vi "Main.vi"(11 "Module Admin":refnum<class "Delacor_lib_QMH_Module Admin.lvclass">) -> ()   [LabVIEW 2023, in "AutoPV.lvlib"]
doc: "This template is based off of the Queued Message Handler design pattern and the Queued Message Handler project template that ships with LabVIEW.\n\nThe main difference is that the queue is private to this module and communication between modules is performed via Broadcast and Request events.\n\nRequest events are wrapped in public API methods and are handled in the Event Handling Loop (EHL) of this VI. Any module can register for Broadcast events sent by this module. The EHL generates messages based on user interface actions.\n\nThe Message Handling Loop (MHL) processes messages generated by the EHL, or by other messages. The messages are string values, so new messages can be added easily to the Message Cases case structure in the MHL. Each message cluster can also provide an optional value for Message Data, which is a variant that can be converted to whatever message-specific data is required.\n_____\nBased on DQMH Project Template 6.1.0.94."
uses:
  AutoPV.lvlib
  <vilib>/Delacor/Delacor QMH/Libraries/Module Admin_class/Delacor_lib_QMH_Module Admin.lvclass
  Module Data--cluster.ctl
  <vilib>/ActorFramework/Message Enqueuer/Message Enqueuer.lvclass
  Drive/Pump_Data_Type.ctl
  Initial Data/InitalData Type.ctl
  Stop Argument--cluster.ctl
  <vilib>/Delacor/Delacor QMH/Libraries/Message Queue_class/Delacor_lib_QMH_Message Queue.lvclass/Delacor_lib_QMH_Message Queue.ctl
  <vilib>/Delacor/Delacor QMH/Libraries/Module Admin_class/Delacor_lib_QMH_Module Admin.lvclass/Delacor_lib_QMH_Module Admin.ctl
  Write_Dot Argument--cluster.ctl
  Update List UI Argument--cluster.ctl
  SubPanel Argument--cluster.ctl
  <vilib>/Utility/miscctls.llb/LVPointTypeDef.ctl
  Param_SL.ctl
  <vilib>/Delacor/Delacor QMH/Libraries/Message Queue_class/Delacor_lib_QMH_Enqueue Message (Single).vi
  <vilib>/Delacor/Delacor QMH/Libraries/Module Admin_class/Delacor_lib_QMH_Get External Launch.vi
  <vilib>/Analysis/baseanly.llb/Mean (DBL).vi
  <vilib>/Utility/file.llb/Read Delimited Spreadsheet (string).vi
  <vilib>/Utility/file.llb/Write Delimited Spreadsheet (string).vi
  <vilib>/Utility/error.llb/Error Cluster From Error Code.vi
  <vilib>/ErrorRing/Error Ring.xnode
  <vilib>/Delacor/Delacor QMH/Libraries/Message Queue_class/Delacor_lib_QMH_Message Queue.lvclass
  SFC/SFC.lvlib
  <vilib>/Kortex/Actor Planer/Actor Planer.lvlib
  <vilib>/Analysis/NI_AALBase.lvlib
  Drive/Drive.lvlib
  <vilib>/Utility/sysdir.llb/System Directory Type.ctl
  <vilib>/Utility/config.llb/NI_LVConfig.lvlib
  Initial Data/Initial Data.lvlib
  Dispatcher/Dispatcher.lvlib
panel:
  in  "Add 2":bool
  in  "Delete 2":bool
  in  "Save 2":bool
  in  "Load 2":bool
  in  "Архив экспериментов 2":bool
  in  "Add":bool
  in  "Pressure_edit":dbl=0.1 caption="Рредакт." min=0.1 max=99.99 format="%#.3f МПа"
  in  "Delete":bool
  in  "Save":bool
  in  "Load":bool
  in  "Pressure_List":i32(listbox) caption="Рзад, МПа"
  in  "Start":bool
  out "Time 2":dbl caption="Время отстоя" min=0.0 max=9999.0 format="%d сек."
  out "Mix_RPM 2":dbl=0.1 caption="Обороты мешалки" min=-1500.0 max=1500.0 format="%#.1f об\\мин"
  out "Stab_dP 2":dbl=0.1 caption="Стабилизация" min=0.1 max=20.0 format="%#.3f МПа"
  out "N 2":u32=1 caption="Текущая ступень" min=1 max=9999
  out "Stab_Time 2":dbl caption="Время перемешивания" min=0.0 max=9999.0 format="%d сек."
  out "dP 2":dbl=0.1 caption="Уставка давления" min=0.1 max=20.0 format="%#.2f МПа"
  out "P0 2":dbl=1.0 caption="Текущее давление" min=1.0 max=99.0 format="%#.2f МПа"
  in  "Time":dbl caption="Время отстоя" min=0.0 max=9999.0 format="%#.1f сек."
  in  "Mix_RPM":dbl=0.1 caption="Обороты мешалки" min=-1500.0 max=1500.0 format="%#.1f об\\мин"
  in  "Stab_dP":dbl=0.1 caption="Условие стабилизации" min=0.001 max=20.0 format="%#.3f МПа"
  in  "N":u32=1 caption="Кол-во ступеней" min=1 max=9999
  in  "Stab_Time":dbl caption="Время перемешивания" min=0.0 max=9999.0 format="%#.1f сек."
  out "relative seconds":dbl format="%_19f"
  in  "dP":dbl=0.1 caption="Шаг по давлению" min=0.01 max=20.0 format="%#.2f МПа"
  in  "P0":dbl=1.0 caption="Начальное давление" min=1.0 max=99.0 format="%#.2f МПа"
  in  "Pop-Out Tool 2":bool
  in  "Pop-Out Tool":bool
  out "PV-График":T1(graph)
  out "error out":errorcluster
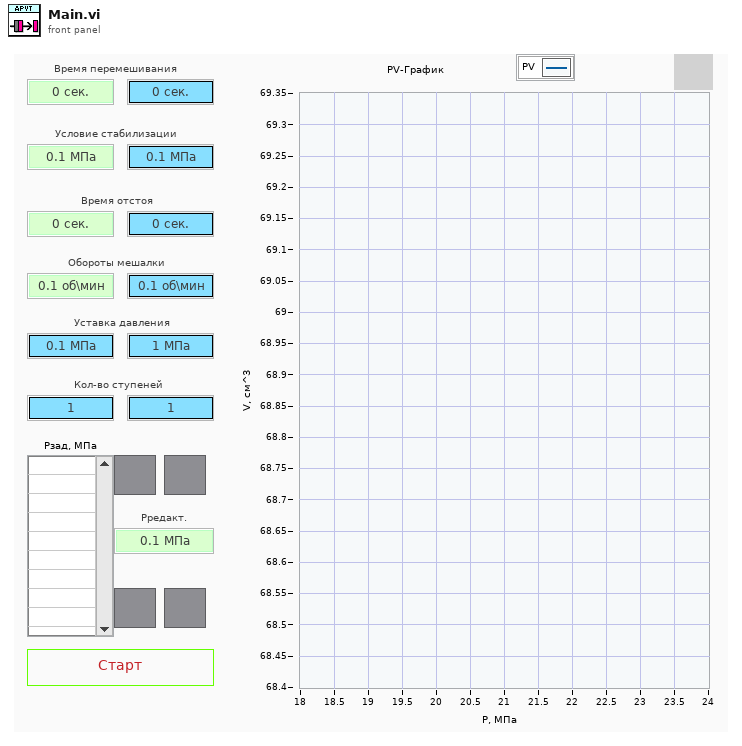
[diagram p1: front panel]
types:
  T1 = cluster{"Array - Dots":dbl[], "Array - Dots":dbl[]}
  T2 = typedef "Heat UI.lvlib/Broadcast Events--cluster.ctl" = cluster{"Module Did Init":refnum<user-event>, "Status Updated":refnum<user-event>, "Error Reported":refnum<user-event>, "Module Did Stop":refnum<user-event>, "Update Module Execution Status":refnum<user-event>, "T Data":refnum<user-event>, "Temp array":refnum<user-event>}
  T3 = typedef "Dispatcher.lvlib/Broadcast Events--cluster.ctl" = cluster{"Module Did Init":refnum<user-event>, "Status Updated":refnum<user-event>, "Error Reported":refnum<user-event>, "Module Did Stop":refnum<user-event>, "Update Module Execution Status":refnum<user-event>}
  T4 = typedef "Initial Data.lvlib/Broadcast Events--cluster.ctl" = cluster{"Module Did Init":refnum<user-event>, "Status Updated":refnum<user-event>, "Error Reported":refnum<user-event>, "Module Did Stop":refnum<user-event>, "Update Module Execution Status":refnum<user-event>, "Data":refnum<user-event>}
  T5 = typedef "Drive.lvlib/Broadcast Events--cluster.ctl" = cluster{"Module Did Init":refnum<user-event>, "Status Updated":refnum<user-event>, "Error Reported":refnum<user-event>, "Module Did Stop":refnum<user-event>, "Update Module Execution Status":refnum<user-event>, "Pump_Data":refnum<user-event>, "Rotate Data":refnum<user-event>, "Pump2 data":refnum<user-event>}
  T6 = typedef "AutoPV.lvlib/Request Events--cluster.ctl" = cluster{"Stop Module":refnum<user-event>, "Show Panel":refnum<user-event>, "Hide Panel":refnum<user-event>, "Get Module Execution Status":refnum<user-event>, "Show Diagram":refnum<user-event>, "Write_Dot":refnum<user-event>, "Update List UI":refnum<user-event>, "SubPanel":refnum<user-event>}
  T7 = typedef "SFC.lvlib/Control TypeDef.ctl" = cluster{"queue":refnum<queue>, "error":errorcluster, "Step":T8, "Algorythm":T8[]}
  T8 = typedef "SFC.lvlib/Step TypeDef.ctl" = cluster{"Name":string, "Timeout":dbl}
  T9 = typedef "AutoPV.lvlib/Module Data--cluster.ctl" = cluster{"Plan Enqueuer":refnum<class "Message Enqueuer.lvclass">, "Array P":dbl[], "Pump_data":T10, "Array - Dots":dbl[][], "Исходные данные":T11, "Temp array":dbl[], "Pressure_List ref":refnum<vi>, "Table select":i32, "PV_N":i32, "PV_N ref":refnum<vi>, "N ref":refnum<vi>, "Subpanel Ref":refnum<vi>}
  T10 = typedef "Drive.lvlib/Pump_Data_Type.ctl" = cluster{"Pressure PV":dbl, "Flow PV":dbl, "Volume PV":dbl, "Position_MM":dbl, "Volume corrected":dbl, "mix rpm":dbl}
  T11 = typedef "Initial Data.lvlib/InitalData Type.ctl" = cluster{"Дата":string, "Время":string, "Месторождение":string, "Пласт":string, "Скважина":string}
  T12 = enum32{"Invalid", "Standard", "Closed", "Hidden", "Minimized", "Maximized"}
  T13 = enum32{"invalid lock state", "Not Locked", "Locked (No Password)", "Password-protected"}
  T14 = typedef "AutoPV.lvlib/Stop Argument--cluster.ctl" = cluster{"Origin":string, "Exit via Stop Module Req?":bool, "Wait for Module to stop?":bool}
  T15 = typedef "AutoPV.lvlib/Write_Dot Argument--cluster.ctl" = cluster{"Clean?":bool, "Finish?":bool}
  T16 = typedef "AutoPV.lvlib/Update List UI Argument--cluster.ctl" = cluster{"Boolean":bool}
  T17 = typedef "AutoPV.lvlib/SubPanel Argument--cluster.ctl" = cluster{"Sub Panel":refnum<vi>}
  T18 = typedef "AutoPV.lvlib/Param_SL.ctl" = cluster{"P0":dbl, "dP":dbl, "Stab_Time":dbl, "N":u32, "Stab_dP":dbl, "Mix_RPM":dbl, "Time":dbl, "Item Names":string[]}
  T19 = typedef "LVPointTypeDef.ctl" = cluster{"Horizontal":i16, "Vertical":i16}
  T20 = typedef "NI_LVConfig.lvlib/Config Data RefNum.ctl" = refnum<k1>
  T21 = typedef "System Directory Type.ctl" = i32
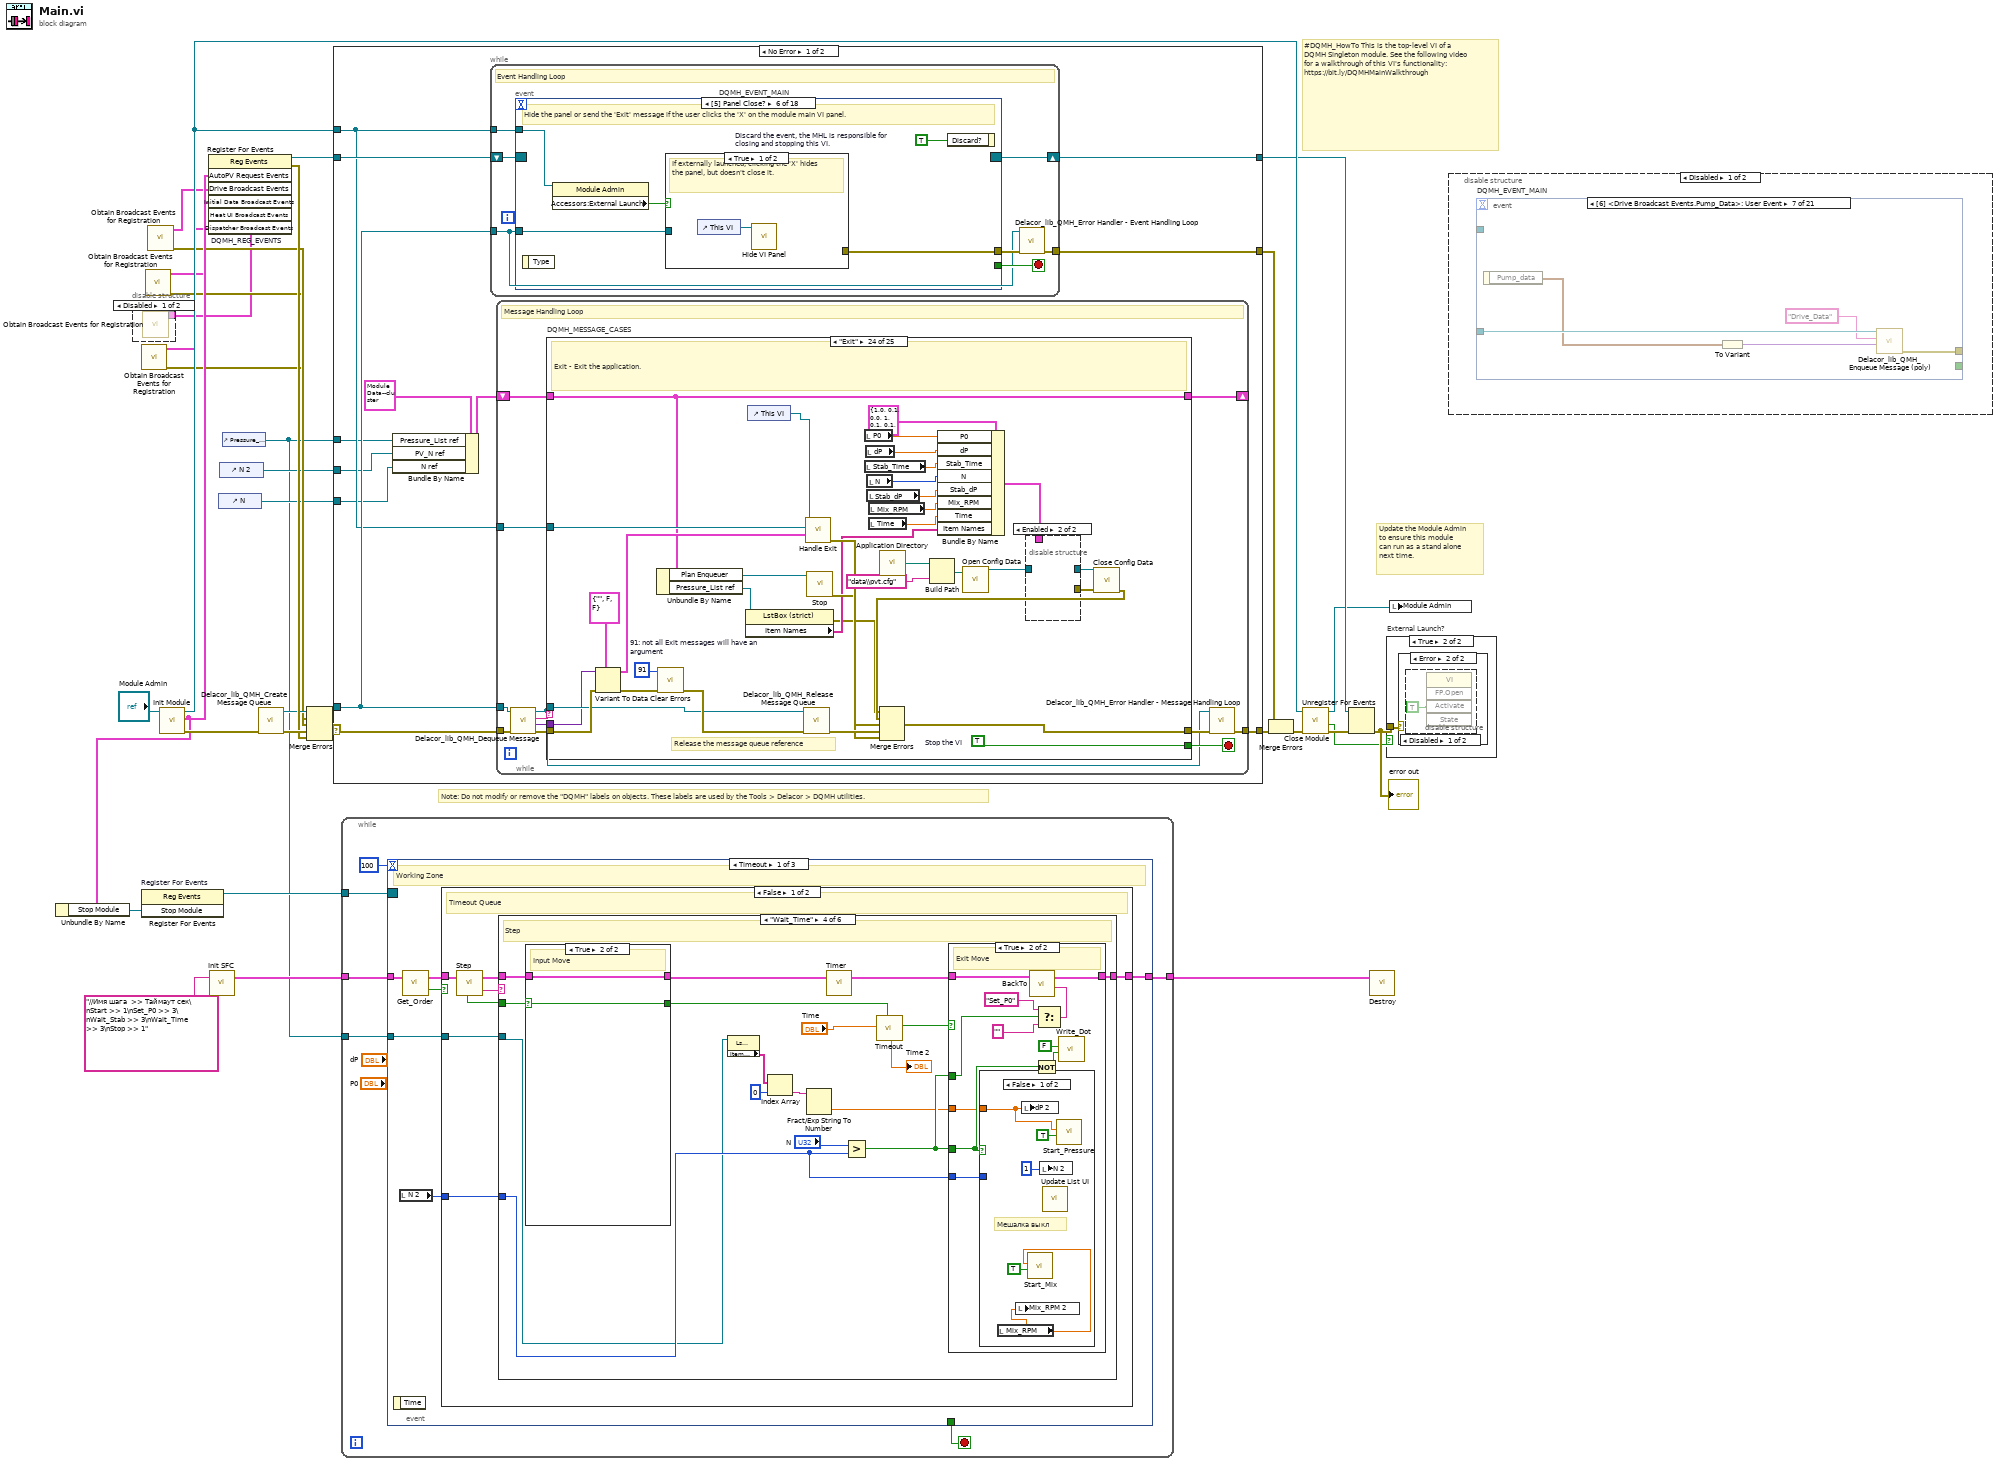
[diagram p0: block diagram]
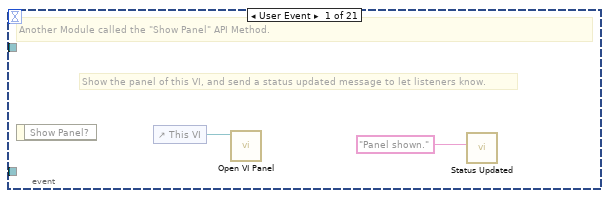
[diagram p2: hidden frame]
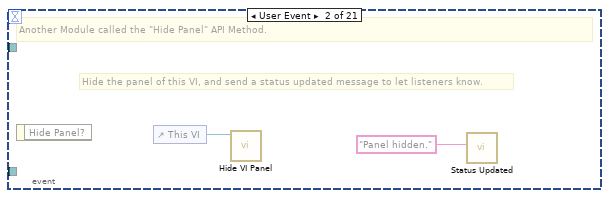
[diagram p3: hidden frame]
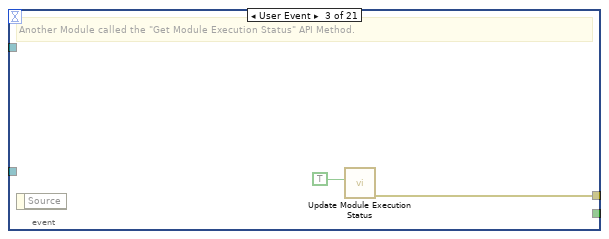
[diagram p4: hidden frame]
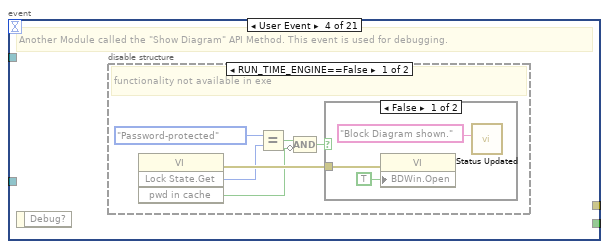
[diagram p5: hidden frame]
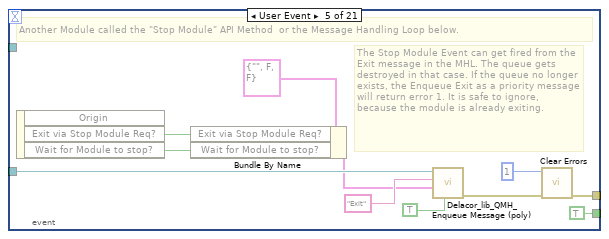
[diagram p8: hidden frame]
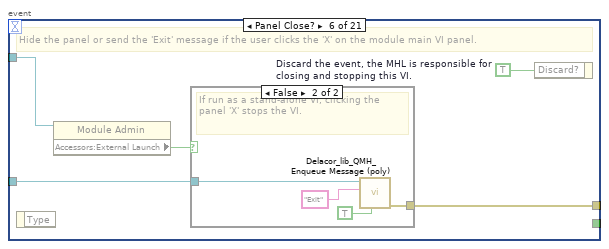
[diagram p9: hidden frame]
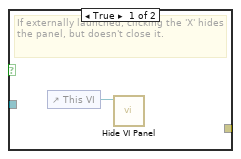
[diagram p10: hidden frame]
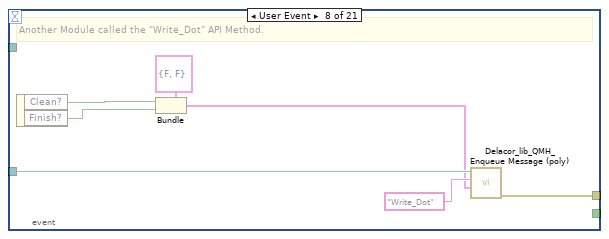
[diagram p11: hidden frame]
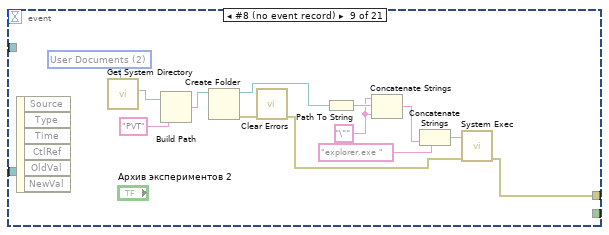
[diagram p12: hidden frame]
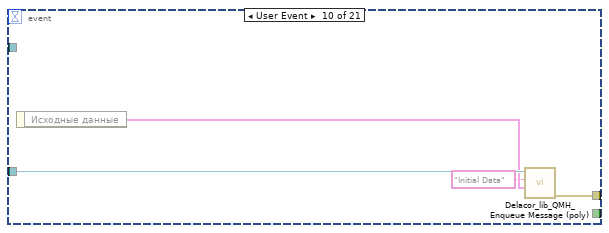
[diagram p13: hidden frame]
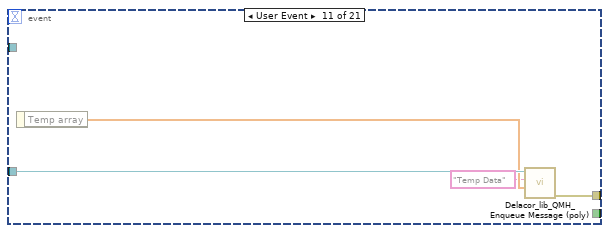
[diagram p14: hidden frame]
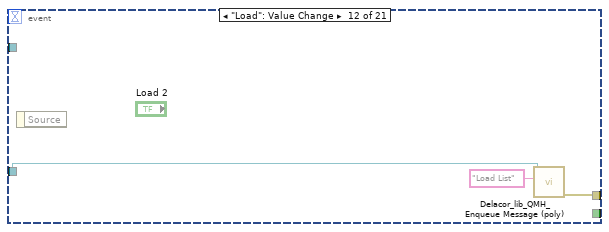
[diagram p15: hidden frame]
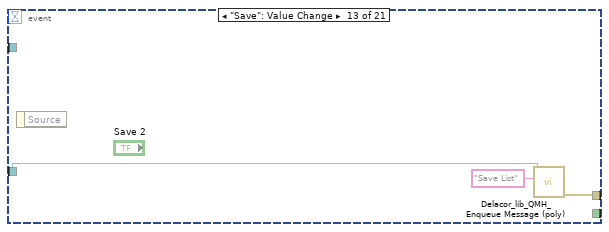
[diagram p16: hidden frame]
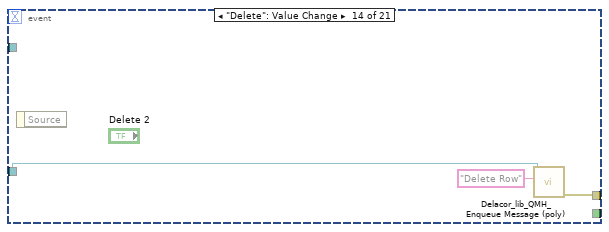
[diagram p17: hidden frame]
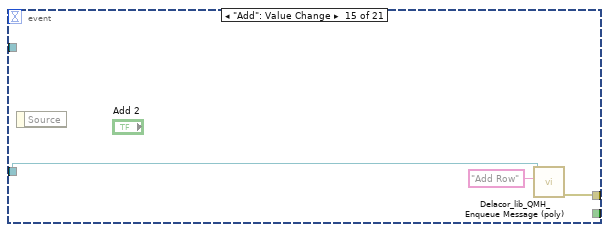
[diagram p18: hidden frame]
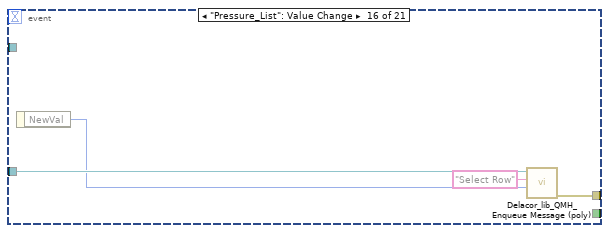
[diagram p19: hidden frame]
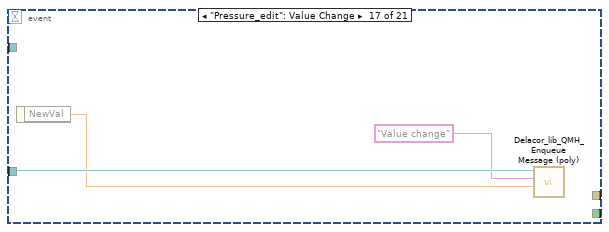
[diagram p20: hidden frame]
diagram:
  # "#DQMH_HowTo This is the top-level VI of a DQMH Singleton module. See the following video for a walkthrough of this VI's functionality: https://bit.ly/DQMHMainWalkthrough"
  # "Note: Do not modify or remove the \"DQMH\" labels on objects. These labels are used by the Tools > Delacor > DQMH utilities."
  # "Update the Module Admin to ensure this module can run as a stand alone next time."
  n1 = disable-structure shown="Disabled" {
    disable-tunnel: [w33 _] -> w6
    frame Disabled {
      n2 = call "Obtain Broadcast Events for Registration.vi"() -> ("Heat UI Broadcast Events"=w33:T2)  [unwired: 9 in, 2 out]
    }
    frame Enabled {
    }
  }
  n3 = call "Obtain Broadcast Events for Registration.vi"() -> ("error out"=w1:errorcluster, "Dispatcher Broadcast Events"=w2:T3)  [unwired: 9 in, 1 out]
  n4 = call "Obtain Broadcast Events for Registration.vi"() -> ("error out"=w7:errorcluster, "Initial Data Broadcast Events"=w8:T4)  [unwired: 9 in, 1 out]
  n5 = call "Obtain Broadcast Events for Registration.vi"() -> ("error out"=w9:errorcluster, "Drive Broadcast Events"=w10:T5)  [unwired: 9 in, 1 out]
  n6 = call "Init Module.vi"("Singleton Module Admin in"="Module Admin") -> ("error out"=w31:errorcluster, "AutoPV Request Events"=w12:T6, "Singleton Module Admin out"=w23:refnum<class "Delacor_lib_QMH_Module Admin.lvclass">)  [unwired: 8 in]
  n7 = Unbundle By Name(w12) -> ("Stop Module"=w11:refnum<user-event>)
  n8 = register-events "Register For Events"(w11) -> (reference out=w16:refnum<event-registration>)  [unwired: 2 in, 1 out]
  n9 = register-events "DQMH_REG_EVENTS"(w12, w10, w8, w6, w2) -> (reference out=w21:refnum<event-registration>, error out=w24:errorcluster)  [unwired: 2 in]
  n10 = call "Init SFC.vi"("Algo"="//Имя шага  >> Таймаут сек\nStart >> 1\nSet_P0 >> 3\nWait_Stab >> 3\nWait_Time >> 3\nStop >> 1") -> ("Control"=w15:T7)  [unwired: 18 in]
  n11 = control-ref of="N"() -> (w4:refnum<vi>)
  n12 = control-ref of="N 2"() -> (w5:refnum<vi>)
  n13 = control-ref of="Pressure_List"() -> (w3:refnum<vi>)
  n14 = call <vilib>:"Delacor_lib_QMH_Create Message Queue.vi"("error in"=w31) -> ("error out"=w26:errorcluster, "Message Queue"=w20:refnum<class "Delacor_lib_QMH_Message Queue.lvclass">)  [unwired: 9 in]
  n15 = Merge Errors(w1, w7, w9, w26, w24) -> (w25:errorcluster)
  n16 = case shown="No Error" w25 {
    selector: w25 -> [w43 w492]
    tunnel: [w45 w491] -> w32
    tunnel: [w42 w497] -> w22
    tunnel: w21 -> [w40 w497]
    tunnel: w20 -> [w39 w490]
    tunnel: [w44 _] -> w29
    tunnel: w23 -> [w38 w493]
    tunnel: w3 -> [w36 _]
    tunnel: w5 -> [w35 _]
    tunnel: w4 -> [w34 _]
    frame No Error {
      n17 = Bundle By Name(cluster=T9 {"Plan Enqueuer"=refnum, "Array P"=[], "Pump_data"={"Pressure PV"=0.0, "Flow PV"=0.0, "Volume PV"=0.0, "Position_MM"=0.0, "Volume corrected"=0.0, "mix rpm"=0.0}, "Array - Dots"=[], "Исходные данные"={"Дата"="", "Время"="", "Месторождение"="", "Пласт"="", "Скважина"=""}, "Temp array"=[], "Pressure_List ref"=refnum, "Table select"=0, "PV_N"=0, "PV_N ref"=refnum, "N ref"=refnum, "Subpanel Ref"=refnum} ("Data Cluster"), "Pressure_List ref"=w36, "PV_N ref"=w35, "N ref"=w34) -> (w37:T9)
      n18 = while {
        tunnel: w39 -> [w46]
        shift-right: [w49] -> w42
        shift-left: w40 -> [w50]
        tunnel: [w51] -> w44
        tunnel: w38 -> [w47]
        stop <- w48 stop-if-true
        # "Event Handling Loop"
        n19 = event "DQMH_EVENT_MAIN" shown="[5] Panel Close?" {
          selector: w50 -> [_ _ _ _ _ _ _ _ _ _ _ _ _ _ _ _ _ _]
          dyn-events: [_ _ _ _ _ _ _ _ _ _ _ _ _ _ _ _ _ _] -> w49
          timeout: _ -> [_ _ _ _ _ _ _ _ _ _ _ _ _ _ _ _ _ _]
          tunnel: [_ _ _ _ TRUE ("Discard?") _ _ _ _ _ _ _ _ _ _ _ _ _] -> w48
          tunnel: w46 -> [_ _ _ _ w76 w83 w94 w102 w106 w108 w111 w114 w117 w121 w125 w131 w137 w138]
          tunnel: [_ _ w60 _ w79 w85 w95 w97 w103 w109 w112 w115 w118 w122 _ w126 w132 w139] -> w52
          tunnel: w47 -> [_ _ _ _ _ w82 _ _ _ _ _ _ _ _ _ _ _ _]
          event User Event {
            # "Show the panel of this VI, and send a status updated message to let listeners know."
            # "Another Module called the \"Show Panel\" API Method."
            n20 = event-data() -> ()  [unwired: 1 in, 1 out]
            n21 = control-ref of="This VI"() -> (w54:refnum<vi>)
            n22 = call "Open VI Panel.vi"("VI"=w54) -> ()  [unwired: 10 in, 1 out]
            n23 = call "Status Updated.vi"("Status"="Panel shown." ("format string")) -> ()  [unwired: 10 in, 1 out]
          }
          event User Event {
            # "Hide the panel of this VI, and send a status updated message to let listeners know."
            # "Another Module called the \"Hide Panel\" API Method."
            n24 = event-data() -> ()  [unwired: 1 in, 1 out]
            n25 = control-ref of="This VI"() -> (w57:refnum<vi>)
            n26 = call "Hide VI Panel.vi"("VI"=w57) -> ()  [unwired: 10 in, 1 out]
            n27 = invoke class="VI" method="FP.Open"(reference=w57, "Activate"=FALSE ("Activate?"), "State"=T12."Closed") -> ()  [unwired: 2 in, 5 out]
            n28 = call "Status Updated.vi"("Status"="Panel hidden." ("format string")) -> ()  [unwired: 10 in, 1 out]
          }
          event User Event {
            # "Another Module called the \"Get Module Execution Status\" API Method."
            n29 = event-data() -> ()  [unwired: 1 in, 1 out]
            n30 = call "Update Module Execution Status.vi"("Running?"=TRUE) -> ("error out"=w60:errorcluster)  [unwired: 10 in]
          }
          event User Event {
            # "Another Module called the \"Show Diagram\" API Method. This event is used for debugging."
            n31 = event-data() -> ()  [unwired: 1 in, 1 out]
            n32 = disable-structure shown="RUN_TIME_ENGINE==False" {
              frame condition #0 (active) {
                # "functionality not available in exe"
                n33 = invoke class="VI" method="Lock State.Get"() -> (error out=w66:errorcluster, "Get Lock State"=w65:T13, "pwd in cache"=w62:bool)  [unwired: 4 in, 1 out]
                n34 = Equal?(x=T13."Password-protected", y=w65) -> (x = y?=w63:bool)
                n35 = Compound Arithmetic op=AND(w63, invert w62) -> (w61:bool)
                n36 = case shown="False" w61 {
                  tunnel: w66 -> [w69 _]
                  frame False {
                    n37 = property class="VI"(error in=w69, "BDWin.Open"=TRUE ("Block Diagram Window:Open")) -> ()  [unwired: 1 in, 2 out]
                    n38 = call "Status Updated.vi"("Status"="Block Diagram shown." ("format string")) -> ()  [unwired: 10 in, 1 out]
                  }
                  frame True {
                    # "Password-protected VI, and the password is not in the cache. Do not show the diagram."
                  }
                }
              }
              frame condition #1 {
              }
            }
          }
          event User Event {
            # "The Stop Module Event can get fired from the Exit message in the MHL. The queue gets destroyed in that case. If the queue no longer exists, the Enqueue Exit as a priority message will return error 1. It is safe to ignore, because the module is already exiting."
            # "Another Module called the \"Stop Module\" API Method  or the Message Handling Loop below."
            n39 = event-data() -> ("Exit via Stop Module Req?"=w72:bool, "Wait for Module to stop?"=w71:bool)  [unwired: 1 in, 1 out]
            n40 = Bundle By Name(cluster=T14 {"Origin"="", "Exit via Stop Module Req?"=FALSE, "Wait for Module to stop?"=FALSE} ("Stop Argument"), "Exit via Stop Module Req?"=w72, "Wait for Module to stop?"=w71) -> (w70:T14)
            n41 = call-poly <vilib>:"Delacor_lib_QMH_Enqueue Message (poly).vi"("Priority Message? (F)"=TRUE, "Message Data"=w70, "Message"="Exit", "Message Queue in"=w76) -> ("error out"=w80:errorcluster)  [unwired: 6 in, 1 out]
            n42 = call <vilib>:"Clear Errors.vi"("error in (no error)"=w80, "specific error code to clear (0: all)"=1) -> ("error out"=w79:errorcluster)  [unwired: 4 in, 1 out]
          }
          event Panel Close? {
            w84 = TRUE  # Discard the event, the MHL is responsible for closing and stopping this VI.
            # "Hide the panel or send the 'Exit' message if the user clicks the 'X' on the module main VI panel."
            n43 = event-data() -> ()  [unwired: 1 in, 1 out]
            n44 = property class="Module Admin"(reference=w82) -> ("Accessors:External Launch"=w81:bool)  [unwired: 1 in, 2 out]
            n45 = case shown="True" w81 {
              tunnel: w83 -> [_ w89]
              tunnel: [_ w90] -> w85
              frame True {
                # "If externally launched, clicking the 'X' hides the panel, but doesn't close it."
                n46 = control-ref of="This VI"() -> (w86:refnum<vi>)
                n47 = call "Hide VI Panel.vi"("VI"=w86) -> ()  [unwired: 10 in, 1 out]
              }
              frame False {
                # "If run as a stand-alone VI, clicking the panel 'X' stops the VI."
                n48 = call-poly <vilib>:"Delacor_lib_QMH_Enqueue Message (poly).vi"("Priority Message? (F)"=TRUE, "Message"="Exit", "Message Queue in"=w89) -> ("error out"=w90:errorcluster)  [unwired: 7 in, 1 out]
              }
            }
            n49 = event-data("Discard?"=w84) -> ()  [unwired: 1 in, 1 out]
          }
          event User Event {
            n50 = event-data() -> ("Pump_data"=w93:T10)  [unwired: 1 in]
            n51 = To Variant(anything=w93) -> (Variant=w91:variant)
            n52 = call-poly <vilib>:"Delacor_lib_QMH_Enqueue Message (poly).vi"("Message Data"=w91, "Message"="Drive_Data", "Message Queue in"=w94) -> ("error out"=w95:errorcluster)  [unwired: 7 in, 1 out]
          }
          event User Event {
            # "Another Module called the \"Write_Dot\" API Method."
            n53 = event-data() -> ("Clean?"=w98:bool, "Finish?"=w96:bool)  [unwired: 1 in]
            n54 = Bundle(cluster=T15 {"Clean?"=FALSE, "Finish?"=FALSE} ("Write_Dot Argument"), "Clean?"=w98, "Finish?"=w96) -> (w99:T15)
            n55 = call-poly <vilib>:"Delacor_lib_QMH_Enqueue Message (poly).vi"("Message Data"=w99, "Message"="Write_Dot", "Message Queue in"=w102) -> ("error out"=w97:errorcluster)  [unwired: 7 in, 1 out]
          }
          event User Event {
            n56 = event-data() -> ("Исходные данные"=w105:T11)  [unwired: 1 in]
            n57 = call-poly <vilib>:"Delacor_lib_QMH_Enqueue Message (poly).vi"("Message Data"=w105, "Message"="Initial Data", "Message Queue in"=w106) -> ("error out"=w103:errorcluster)  [unwired: 7 in, 1 out]
          }
          event "Load": Value Change {
            n58 = event-data() -> ()  [unwired: 1 in, 1 out]
            n59 = call-poly <vilib>:"Delacor_lib_QMH_Enqueue Message (poly).vi"("Message"="Load List", "Message Queue in"=w108) -> ("error out"=w109:errorcluster)  [unwired: 8 in, 1 out]
          }
          event "Save": Value Change {
            n60 = event-data() -> ()  [unwired: 1 in, 1 out]
            n61 = call-poly <vilib>:"Delacor_lib_QMH_Enqueue Message (poly).vi"("Message"="Save List", "Message Queue in"=w111) -> ("error out"=w112:errorcluster)  [unwired: 8 in, 1 out]
          }
          event "Delete": Value Change {
            n62 = event-data() -> ()  [unwired: 1 in, 1 out]
            n63 = call-poly <vilib>:"Delacor_lib_QMH_Enqueue Message (poly).vi"("Message"="Delete Row", "Message Queue in"=w114) -> ("error out"=w115:errorcluster)  [unwired: 8 in, 1 out]
          }
          event "Add": Value Change {
            n64 = event-data() -> ()  [unwired: 1 in, 1 out]
            n65 = call-poly <vilib>:"Delacor_lib_QMH_Enqueue Message (poly).vi"("Message"="Add Row", "Message Queue in"=w117) -> ("error out"=w118:errorcluster)  [unwired: 8 in, 1 out]
          }
          event "Pressure_List": Value Change {
            n66 = event-data() -> ("NewVal"=w120:i32)  [unwired: 1 in]
            n67 = call-poly <vilib>:"Delacor_lib_QMH_Enqueue Message (poly).vi"("Message Data"=w120, "Message"="Select Row", "Message Queue in"=w121) -> ("error out"=w122:errorcluster)  [unwired: 7 in, 1 out]
          }
          event "Pressure_edit": Value Change {
            n68 = event-data() -> ("NewVal"=w124:dbl)  [unwired: 1 in]
            n69 = call-poly <vilib>:"Delacor_lib_QMH_Enqueue Message (poly).vi"("Message Data"=w124, "Message"="Value change", "Message Queue in"=w125) -> ()  [unwired: 7 in, 2 out]
          }
          event User Event {
            # "Another Module called the \"Update List UI\" API Method."
            n70 = event-data() -> ("Boolean"=w127:bool)  [unwired: 1 in]
            n71 = Bundle(cluster=T16 {"Boolean"=FALSE} ("Update List UI Argument"), "Boolean"=w127) -> (w128:T16)
            n72 = call-poly <vilib>:"Delacor_lib_QMH_Enqueue Message (poly).vi"("Message Data"=w128, "Message"="Update List UI", "Message Queue in"=w131) -> ("error out"=w126:errorcluster)  [unwired: 7 in, 1 out]
          }
          event User Event {
            # "Another Module called the \"SubPanel\" API Method."
            n73 = event-data() -> ("Sub Panel"=w133:refnum<vi>)  [unwired: 1 in]
            n74 = Bundle(cluster=T17 {"Sub Panel"=refnum} ("SubPanel Argument"), "Sub Panel"=w133) -> (w134:T17)
            n75 = call-poly <vilib>:"Delacor_lib_QMH_Enqueue Message (poly).vi"("Message Data"=w134, "Message"="SubPanel", "Message Queue in"=w137) -> ("error out"=w132:errorcluster)  [unwired: 7 in, 1 out]
          }
          event "Pop-Out Tool": Value Change {
            n76 = event-data() -> ()  [unwired: 1 in, 2 out]
            n77 = call-poly <vilib>:"Delacor_lib_QMH_Enqueue Message (poly).vi"("Message"="Window", "Message Queue in"=w138) -> ("error out"=w139:errorcluster)  [unwired: 8 in, 1 out]
          }
        }
        n78 = call-dynamic "Delacor_lib_QMH_Error Handler - Event Handling Loop.vi"("error in"=w52, "Message Queue in"=w46) -> ("dup error in"=w51:errorcluster)  [unwired: 8 in, 1 out]
      }
      n79 = while {
        tunnel: w39 -> [w143]
        shift-right: [w147] -> _
        shift-left: w37 -> [w148]
        tunnel: w43 -> [w151]
        tunnel: [w149] -> w45
        tunnel: w38 -> [w141]
        stop <- w146 stop-if-true
        # "Message Handling Loop"
        n80 = call-dynamic "Delacor_lib_QMH_Dequeue Message.vi"("error in"=w151, "Message Queue in"=w143) -> ("error out"=w150:errorcluster, "Message Data"=w144:variant, "Message"=w145:string, "Message Queue out"=w142:refnum<class "Delacor_lib_QMH_Message Queue.lvclass">)  [unwired: 6 in]
        n81 = case "DQMH_MESSAGE_CASES" shown="\"Exit\"" w145 {
          selector: w145 -> [_ _ _ _ _ _ _ _ _ _ _ _ _ _ _ _ _ _ _ _ _ _ _ _ w477]
          tunnel: w142 -> [w161 _ w191 _ _ _ _ _ _ _ _ _ _ _ _ _ _ w370 _ _ _ _ w422 w465 _]
          tunnel: w150 -> [w185 w188 w205 w219 w227 w243 w256 w262 w273 w276 w285 w292 w300 w309 w316 w323 w340 w375 w392 w405 w407 w412 w429 w471 w479]
          tunnel: [w171 w188 w193 w214 w222 w240 w252 w261 w266 w275 w284 w291 w299 w308 w315 w322 w339 w382 w394 w404 w407 w411 w425 w468 w480] -> w152
          tunnel: w148 -> [w156 w187 w197 w215 w223 w238 w250 w258 w272 w274 w283 w290 w298 w306 w314 w321 w324 w381 w393 w400 w406 w409 w424 w457 w478]
          tunnel: [w176 w187 w199 w216 w224 w238 w253 w257 w264 w274 w283 w289 w297 w306 w314 w321 w324 w381 w389 w400 w406 w409 w424 w457 w478] -> w147
          tunnel: [_ _ _ _ _ _ _ _ _ _ _ _ _ _ _ _ _ _ _ _ _ _ _ w464 _] -> w146
          tunnel: w144 -> [_ _ w203 w217 w225 w241 w254 w260 w270 _ _ _ _ _ _ _ _ w374 w391 _ _ _ w423 w463 _]
          tunnel: w141 -> [w177 _ _ _ _ _ _ _ _ _ _ _ _ _ _ _ _ _ _ _ _ _ w421 w458 _]
          frame "Initialize" {
            w164 = T19 {"Horizontal"=0, "Vertical"=0} ("Origin")
            # "Initialize - Any operation that needs to be done before the module can receive messages. Synchronize Caller Events.vi will inform Start Module.vi that the module has launched and is ready to receive messages. Module Did Init.vi will broadcast that the module initialized."
            n82 = call "Synchronize Caller Events.vi"("error in (no error)"=w185, "Singleton Module Admin in"=w177) -> ("error out"=w184:errorcluster, "Singleton Module Admin out"=w173:refnum<class "Delacor_lib_QMH_Module Admin.lvclass">)  [unwired: 8 in]
            n83 = Unbundle By Name(w156) -> ("Pressure_List ref"=w155:refnum<vi>)
            n84 = property class="Module Admin"(reference=w173) -> ("Accessors:External Launch"=w181:bool)  [unwired: 1 in, 2 out]
            n85 = call <vilib>:"Start.vi"("DQMH Queue"=w161) -> ("error out"=w170:errorcluster, "Plan Enqueuer"=w169:refnum<class "Message Enqueuer.lvclass">)  [unwired: 9 in]
            n86 = property class="LstBox (strict)"(reference=w155, "Value"=-1) -> (error out=w154:errorcluster)  [unwired: 1 in, 1 out]
            n87 = Select(t=T12."Hidden" ("State"), s=w181, f=T12."Standard" ("State")) -> (s? t:f=w178:T12)
            n88 = call <vilib>:"Add Event.vi"("Continius? (F)"=TRUE, "Timeout (1 sec)"=1.0, "error in"=w170, "Action"="Stab" ("Message"), "Plan Enqueuer"=w169) -> ("error out"=w167:errorcluster, "Plan Enqueuer out"=w168:refnum<class "Message Enqueuer.lvclass">)  [unwired: 4 in, 1 out]
            n89 = property class="VI"("Front Panel.Title"="PV-кривая" ("Front Panel Window:Title")) -> (reference out=w182:refnum<vi>, error out=w186:errorcluster)  [unwired: 2 in]
            n90 = call "Module Name--constant.vi"() -> ("Module Name"=w174:string)  [unwired: 11 in]
            n91 = invoke class="VI" method="FP.Open"(reference=w182, error in=w186, "State"=w178) -> ()  [unwired: 2 in, 5 out]
            n92 = call "Module Did Init.vi"("error in (no error)"=w184, "Initialized?"=TRUE, "Origin"=w174) -> ("error out"=w183:errorcluster)  [unwired: 8 in]
            n93 = property on="Pane" class="Pane"("Position"=w164) -> ()  [unwired: 2 in, 2 out]
            n94 = property on="Pane 2" class="Pane"("Position"=w164) -> ()  [unwired: 2 in, 2 out]
            n95 = call-poly <vilib>:"Delacor_lib_QMH_Enqueue Message (poly).vi"("Message"="Load", "Message Queue in"=w161) -> ("error out"=w162:errorcluster)  [unwired: 8 in, 1 out]
            n96 = Merge Errors(w162, w167, w183, w154) -> (w171:errorcluster)
            n97 = Bundle By Name(cluster=w156, "Plan Enqueuer"=w168, "Table select"=-1, "PV_N"=0) -> (w176:T9)
            n98 = local write "Pressure_edit"(0.0 ("Pressure_edit")) -> ()
          }
          frame "---Module Specific---" {
            # "Separator -- The following cases handle messages specific to this Module."
          }
          frame "Write_Dot" {
            n99 = Unbundle By Name(w197) -> ("Array - Dots"=w196:dbl[][], "Pump_data.Pressure PV"=w195:dbl, "Pump_data.Volume corrected"=w194:dbl)
            n100 = Variant To Data(error in=w205, type=T15 {"Clean?"=FALSE, "Finish?"=FALSE} ("Write_Dot Argument"), Variant=w203) -> (data=w201:T15, error out=w204:errorcluster)
            n101 = Unbundle By Name(w201) -> ("Clean?"=w200:bool, "Finish?"=w189:bool)
            n102 = case shown="False" w200 {
              tunnel: [w209 dbl[][] [] ("Array - Dots")] -> w198
              tunnel: w196 -> [w210 _]
              tunnel: w195 -> [w208 _]
              tunnel: w194 -> [w207 _]
              frame False {
                n103 = Build Array(w208, w207) -> (w206:dbl[])
                n104 = Build Array (concatenate)(w210, w206) -> (w209:dbl[][])
              }
              frame True {
              }
            }
            n105 = Bundle By Name(cluster=w197, "Array - Dots"=w198) -> (w199:T9)
            n106 = call-poly <vilib>:"Delacor_lib_QMH_Enqueue Message (poly).vi"("Message Data"=w189, "Message"="Update Graph", "Message Queue in"=w191) -> ("error out"=w192:errorcluster)  [unwired: 7 in, 1 out]
            n107 = Merge Errors(w192, w204) -> (w193:errorcluster)
          }
          frame "Initial Data" {
            n108 = Variant To Data(error in=w219, type=T11 {"Дата"="", "Время"="", "Месторождение"="", "Пласт"="", "Скважина"=""} ("Исходные данные"), Variant=w217) -> (data=w212:T11, error out=w218:errorcluster)
            n109 = Bundle By Name(cluster=w215, "Исходные данные"=w212) -> (w216:T9)
            n110 = Merge Errors(w218) -> (w214:errorcluster)
          }
          frame "Temp Data" {
            n111 = Variant To Data(error in=w227, type=dbl[] [] ("Temp array"), Variant=w225) -> (data=w221:dbl[], error out=w226:errorcluster)
            n112 = Bundle By Name(cluster=w223, "Temp array"=w221) -> (w224:T9)
            n113 = Merge Errors(w226) -> (w222:errorcluster)
          }
          frame "Value change" {
            n114 = Variant To Data(error in=w243, type=0.0 ("NewVal"), Variant=w241) -> (data=w233:dbl, error out=w242:errorcluster)
            n115 = Unbundle By Name(w238) -> ("Pressure_List ref"=w237:refnum<vi>, "Table select"=w235:i32)
            n116 = Number To Fractional String(number=w233, precision (6)=i16 2) -> (F-format string=w232:string)  [unwired: 2 in]
            n117 = property class="LstBox (strict)"(reference=w237) -> (reference out=w231:refnum<vi>, error out=w230:errorcluster, "Item Names"=w236:string[])  [unwired: 1 in]
            n118 = Replace Array Subset(array=w236, new element=w232, index=w235) -> (w229:string[])
            n119 = property class="LstBox (strict)"(reference=w231, error in=w230, "Item Names"=w229) -> (error out=w228:errorcluster)  [unwired: 1 out]
            n120 = Merge Errors(w228, w242) -> (w240:errorcluster)
          }
          frame "Select Row" {
            n121 = Variant To Data(error in=w256, type="Pressure_List", Variant=w254) -> (data=w247:i32, error out=w255:errorcluster)
            n122 = Unbundle By Name(w250) -> ("Pressure_List ref"=w249:refnum<vi>)
            n123 = property class="LstBox (strict)"(reference=w249) -> (error out=w246:errorcluster, "Item Names"=w248:string[])  [unwired: 1 in, 1 out]
            n124 = Bundle By Name(cluster=w250, "Table select"=w247) -> (w253:T9)
            n125 = Index Array(array=w248, index=w247) -> (element=w245:string)
            n126 = Merge Errors(w246, w255) -> (w252:errorcluster)
            n127 = Fract/Exp String To Number(string=w245) -> (number=w244:dbl)  [unwired: 3 in, 1 out]
            n128 = local write "Pressure_edit"(w244) -> ()
          }
          frame "Update List UI" {
            n129 = Variant To Data(error in=w262, type=T16 {"Boolean"=FALSE} ("Update List UI Argument"), Variant=w260) -> (error out=w261:errorcluster)  [unwired: 1 out]
            n130 = call "Update UI List.vi"("Data Cluster"=w258) -> ("Data Cluster 2"=w257:T9)  [unwired: 9 in, 1 out]
          }
          frame "SubPanel" {
            n131 = Variant To Data(error in=w273, type=T17 {"Sub Panel"=refnum} ("SubPanel Argument"), Variant=w270) -> (data=w268:T17, error out=w271:errorcluster)
            n132 = Unbundle By Name(w268) -> ("Sub Panel"=w263:refnum<vi>)
            n133 = control-ref of="This VI"() -> (w267:refnum<vi>)
            n134 = call "Insert SubPanel.vi"("VI Ref"=w267, "Subpanel Ref"=w263) -> ("error out"=w265:errorcluster)  [unwired: 9 in]
            n135 = Bundle By Name(cluster=w272, "Subpanel Ref"=w263) -> (w264:T9)
            n136 = Merge Errors(w265, w271) -> (w266:errorcluster)
          }
          frame "---Copy This Frame---" {
            # "Duplicate this frame when creating new messages.  Change this comment in the duplicated frame to describe this message."
            n137 = Merge Errors(w276) -> (w275:errorcluster)
          }
          frame "Window" {
            # "Duplicate this frame when creating new messages.  Change this comment in the duplicated frame to describe this message."
            n138 = Unbundle By Name(w283) -> ("Subpanel Ref"=w278:refnum<vi>)
            n139 = control-ref of="This VI"() -> (w281:refnum<vi>)
            n140 = invoke class="SubPnl" method="Remove VI"(reference=w278) -> (error out=w279:errorcluster)  [unwired: 2 in, 2 out]
            n141 = invoke class="VI" method="FP.Close"(reference=w281, error in=w279) -> (reference out=w282:refnum<vi>)  [unwired: 1 in, 2 out]
            n142 = invoke class="VI" method="FP.Open"(reference=w282, "State"=T12."Standard") -> (error out=w277:errorcluster)  [unwired: 3 in, 4 out]
            n143 = Merge Errors(w277, w285) -> (w284:errorcluster)
          }
          frame "Add Row" {
            # "Duplicate this frame when creating new messages.  Change this comment in the duplicated frame to describe this message."
            n144 = call "Add row item.vi"("SP P"="Pressure_edit", "Data Cluster in"=w290) -> ("error out"=w288:errorcluster, "Data Cluster out"=w289:T9)  [unwired: 8 in]
            n145 = call "Update List UI.vi"() -> ("error out"=w286:errorcluster)  [unwired: 11 in]
            n146 = Merge Errors(w286, w288, w292) -> (w291:errorcluster)
          }
          frame "Delete Row" {
            # "Duplicate this frame when creating new messages.  Change this comment in the duplicated frame to describe this message."
            n147 = call "Delete row item.vi"("Data Cluster in"=w298) -> ("error out"=w296:errorcluster, "Ok?"=w294:bool, "New P"=w293:dbl, "Data Cluster out"=w297:T9)  [unwired: 7 in]
            n148 = call "Update List UI.vi"() -> ("error out"=w295:errorcluster)  [unwired: 11 in]
            n149 = case shown="True" w294 {
              tunnel: w293 -> [_ w301]
              frame False {
              }
              frame True {
                n150 = local write "Pressure_edit"(w301) -> ()
              }
            }
            n151 = Merge Errors(w295, w296, w300) -> (w299:errorcluster)
          }
          frame "Load List" {
            # "Duplicate this frame when creating new messages.  Change this comment in the duplicated frame to describe this message."
            n152 = Unbundle By Name(w306) -> ("Pressure_List ref"=w305:refnum<vi>)
            n153 = call-poly <vilib>:"Read Delimited Spreadsheet.vi"() -> ("first row"=w302:string[], "error out"=w307:errorcluster)  [unwired: 10 in, 4 out]
            n154 = property class="LstBox (strict)"(reference=w305, "Item Names"=w302) -> (error out=w304:errorcluster)  [unwired: 1 in, 1 out]
            n155 = call "Update List UI.vi"() -> ("error out"=w303:errorcluster)  [unwired: 11 in]
            n156 = Merge Errors(w303, w304, w307, w309) -> (w308:errorcluster)
          }
          frame "Save List" {
            # "Duplicate this frame when creating new messages.  Change this comment in the duplicated frame to describe this message."
            n157 = Unbundle By Name(w314) -> ("Pressure_List ref"=w313:refnum<vi>)
            n158 = property class="LstBox (strict)"(reference=w313) -> (error out=w312:errorcluster, "Item Names"=w311:string[])  [unwired: 1 in, 1 out]
            n159 = call-poly <vilib>:"Write Delimited Spreadsheet.vi"("1D data"=w311) -> ("error out"=w310:errorcluster)  [unwired: 13 in, 1 out]
            n160 = Merge Errors(w312, w310, w316) -> (w315:errorcluster)
          }
          frame "Save Report" {
            # "Duplicate this frame when creating new messages.  Change this comment in the duplicated frame to describe this message."
            n161 = Unbundle By Name(w321) -> ("Исходные данные"=w320:T11, "Temp array"=w318:dbl[], "Array - Dots"=w317:dbl[][])
            n162 = call "Save Report.vi"("Array - Dots"=w317, "Temp array"=w318, "Исходные данные"=w320) -> ("error out"=w319:errorcluster)  [unwired: 8 in]
            n163 = Merge Errors(w319, w323) -> (w322:errorcluster)
          }
          frame "Load" {
            # "Duplicate this frame when creating new messages.  Change this comment in the duplicated frame to describe this message."
            n164 = call <vilib>:"Application Directory.vi"() -> ("Application Directory"=w334:path)
            n165 = Unbundle By Name(w324) -> ("Pressure_List ref"=w327:refnum<vi>)
            n166 = Build Path(base path=w334, name or relative path="data\\pvt.cfg" ("string")) -> (appended path=w332:path)
            n167 = call <vilib>:"Open Config Data.vi"("configuration file path"=w332) -> ("error out"=w335:errorcluster, "file created?"=w338:bool, "refnum"=w337:T20)  [unwired: 8 in]
            n168 = case shown="False" w338 {
              tunnel: w337 -> [w357 w368]
              tunnel: T18 {"P0"=1.0, "dP"=0.1, "Stab_Time"=0.0, "N"=1, "Stab_dP"=0.1, "Mix_RPM"=0.1, "Time"=0.0, "Item Names"=[]} ("Cluster") -> [w354 _]
              tunnel: w335 -> [w345 w367]
              tunnel: [w356 _] -> w331
              tunnel: [w345 w367] -> w330
              tunnel: [w344 w368] -> w329
              tunnel: w327 -> [w343 w365]
              tunnel: [w341 w366] -> w326
              frame False {
                n169 = disable-structure shown="Disabled" {
                  disable-tunnel: w357 -> [w363 _]
                  disable-tunnel: [w362 _] -> w356
                  disable-tunnel: [w361 _] -> w355
                  disable-tunnel: w354 -> [w360 _]
                  disable-tunnel: w345 -> [w359 _]
                  disable-tunnel: [w358 _] -> w344
                  frame Disabled {
                    n170 = call <userlib>:"Read INI Cluster__ogtk.vi"("error in (no error)"=w359, "INI Fomatted Cluster Type"=w360, "refnum"=w363) -> ("error out"=w362:errorcluster, "INI Fomatted Cluster"=w361:variant, "dup refnum"=w358:T20)  [unwired: 4 in, 2 out]
                  }
                  frame Enabled {
                  }
                }
                n171 = Variant To Data(error in=w356, type=w354, Variant=w355) -> (data=w353:T18)  [unwired: 1 out]
                n172 = Unbundle By Name(w353) -> ("Item Names"=w342:string[], "P0"=w352:dbl, "dP"=w351:dbl, "Stab_Time"=w350:dbl, "N"=w349:u32, "Stab_dP"=w348:dbl, "Mix_RPM"=w347:dbl, "Time"=w346:dbl)
                n173 = property class="LstBox (strict)"(reference=w343, "Item Names"=w342) -> (error out=w341:errorcluster)  [unwired: 1 in, 1 out]
                n174 = local write "P0"(w352) -> ()
                n175 = local write "Stab_Time"(w350) -> ()
                n176 = local write "dP"(w351) -> ()
                n177 = local write "N"(w349) -> ()
                n178 = local write "Stab_dP"(w348) -> ()
                n179 = local write "Mix_RPM"(w347) -> ()
                n180 = local write "Time"(w346) -> ()
              }
              frame True {
                n181 = property class="LstBox (strict)"(reference=w365, "Item Names"=string[] []) -> (error out=w366:errorcluster)  [unwired: 1 in, 1 out]
              }
            }
            n182 = call "Update UI List.vi"("error in (no error)"=w326, "Data Cluster"=w324) -> ("error out"=w325:errorcluster)  [unwired: 8 in, 1 out]
            n183 = call <vilib>:"Close Config Data.vi"("error in (no error)"=w330, "refnum"=w329) -> ("error out"=w328:errorcluster)  [unwired: 8 in, 1 out]
            n184 = Merge Errors(w325, w328, w331, w340) -> (w339:errorcluster)
          }
          frame "Update Graph" {
            # "Duplicate this frame when creating new messages.  Change this comment in the duplicated frame to describe this message."
            n185 = Variant To Data(error in=w375, type=FALSE, Variant=w374) -> (data=w369:bool, error out=w372:errorcluster)
            n186 = Unbundle By Name(w381) -> ("Array - Dots"=w380:dbl[][])
            n187 = Transpose 2D Array(2D array=w380) -> (transposed array=w376:dbl[][])
            n188 = Index Array(array=w376) -> (element #1=w379:dbl[], element #2=w378:dbl[])  [unwired: 4 in]
            n189 = case shown="True" w369 {
              tunnel: [_ w385] -> w371
              tunnel: w370 -> [_ w384]
              frame False {
              }
              frame True {
                n190 = call-poly <vilib>:"Delacor_lib_QMH_Enqueue Message (poly).vi"("Message"="Save Report", "Message Queue in"=w384) -> ("error out"=w385:errorcluster)  [unwired: 8 in, 1 out]
              }
            }
            n191 = Bundle(w379, w378) -> (→"PV-График":cluster{dbl[], dbl[]})  [unwired: 1 in]
            n192 = Merge Errors(w371, w372) -> (w382:errorcluster)
          }
          frame "Drive_Data" {
            # "Duplicate this frame when creating new messages.  Change this comment in the duplicated frame to describe this message."
            n193 = Variant To Data(error in=w392, type=T10 {"Pressure PV"=0.0, "Flow PV"=0.0, "Volume PV"=0.0, "Position_MM"=0.0, "Volume corrected"=0.0, "mix rpm"=0.0} ("Pump_data"), Variant=w391) -> (data=w386:T10, error out=w390:errorcluster)
            n194 = Unbundle By Name(w386) -> ("Pressure PV"=→"P0 2":dbl)
            n195 = Bundle By Name(cluster=w393, "Pump_data"=w386) -> (w389:T9)
            n196 = Merge Errors(w390) -> (w394:errorcluster)
          }
          frame "Stab" {
            # "Duplicate this frame when creating new messages.  Change this comment in the duplicated frame to describe this message."
            n197 = Unbundle By Name(w400) -> ("Array P"=w399:dbl[])
            n198 = local read "P0 2"() -> (w402:dbl)
            n199 = local read "dP 2"() -> (w395:dbl)
            n200 = call "Array DBL поддержание размера.vi"("Array size"=20, "New element"=w402, "Array"=w399) -> ("Array out"=w397:dbl[])  [unwired: 8 in]
            n201 = call-poly <vilib>:"Mean.vi"("X"=w397) -> ("mean"=w396:dbl)  [unwired: 1 out]
            n202 = Subtract(x=w395, y=w396) -> (x-y=w398:dbl)
            n203 = Absolute Value(x=w398) -> (abs(x)=→"Stab_dP 2":dbl)
            n204 = Merge Errors(w405) -> (w404:errorcluster)
          }
          frame "---Exit and Error Handling---" {
            # "Separator - The following cases handle errors and exit messages."
          }
          frame "Simulate MHL Error" {
            # "#DQMH_HowTo The 'Simulate MHL Error' button  illustrates how the MHL handles errors. This event is instructional in nature and can be removed."
            # "Simulate an error occurring at the MHL"
            n205 = call "Module Name--constant.vi"() -> ("Module Name"=w408:string)  [unwired: 11 in]
            n206 = xnode "Error Ring"("parameter 0"=w408) -> ("error out"=w410:errorcluster)
            n207 = Merge Errors(w412, w410) -> (w411:errorcluster)
          }
          frame "Error" {
            # "#CodeRecommended - If you ever change the name of this \"Error\" message, you'll need to update the name in the Check Loop Error.vi as well."
            # "#CodeRecommended - If the module is running in standalone mode (External Launch = FALSE), this code will pop up an error dialog and call the 'Exit' message if an error occurs. Add more fine-grained error handling here."
            # "Error - Check the error message data and respond accordingly. This message is sent by the \"Error Handler\" VIs at the end of each loop in this application."
            n208 = property class="Module Admin"(reference=w421) -> ("Accessors:External Launch"=w420:bool)  [unwired: 1 in, 2 out]
            n209 = Variant To Data(error in=w429, type=errorcluster {"status"=FALSE, "code"=0, "source"=""} ("error constant"), Variant=w423) -> (data=w430:errorcluster, error out=w427:errorcluster)
            n210 = call "Error Reported.vi"("Error"=w430) -> ()  [unwired: 10 in, 1 out]
            n211 = case shown="False" w420 {
              tunnel: [w435 _] -> w426
              tunnel: w422 -> [w433 _]
              tunnel: w430 -> [w434 _]
              frame False {
                # "If the module is running standalone, then pop up an error dialog and call the \"Exit\" message."
                n212 = call <vilib>:"Simple Error Handler.vi"("error in (no error)"=w434) -> ()  [unwired: 4 in, 5 out]
                n213 = call-poly <vilib>:"Delacor_lib_QMH_Enqueue Message (poly).vi"("Priority Message? (F)"=TRUE, "Message"="Exit", "Message Queue in"=w433) -> ("error out"=w435:errorcluster)  [unwired: 7 in, 1 out]
              }
              frame True {
                # "If the module was launched externally, calling the Error Reported broadcast VI is the only action performed by the \"Error\" message. The module's caller can then process the error appropriately."
              }
            }
            n214 = Merge Errors(w427, w426) -> (w425:errorcluster)
            n215 = local write "error out"(w425) -> ()
          }
          frame "Exit" {
            w462 = 91  # 91: not all Exit messages will have an argument
            w464 = TRUE  # Stop the VI
            # "Release the message queue reference"
            # "Exit - Exit the application."
            n216 = Variant To Data(error in=w471, type=T14 {"Origin"="", "Exit via Stop Module Req?"=FALSE, "Wait for Module to stop?"=FALSE} ("Stop Argument"), Variant=w463) -> (data=w460:T14, error out=w467:errorcluster)
            n217 = Unbundle By Name(w457) -> ("Plan Enqueuer"=w456:refnum<class "Message Enqueuer.lvclass">, "Pressure_List ref"=w438:refnum<vi>)
            n218 = call <vilib>:"Clear Errors.vi"("error in (no error)"=w467, "specific error code to clear (0: all)"=w462) -> ("error out"=w470:errorcluster)  [unwired: 4 in, 1 out]
            n219 = property class="LstBox (strict)"(reference=w438) -> (error out=w436:errorcluster, "Item Names"=w437:string[])  [unwired: 1 in, 1 out]
            n220 = control-ref of="This VI"() -> (w459:refnum<vi>)
            n221 = call-dynamic "Delacor_lib_QMH_Release Message Queue.vi"("error in"=w470, "Message Queue"=w465) -> ("error out"=w469:errorcluster)  [unwired: 9 in]
            n222 = call "Handle Exit.vi"("Stop Argument"=w460, "Admin in"=w458, "VI reference"=w459) -> ("error out"=w466:errorcluster)  [unwired: 7 in, 1 out]
            n223 = call <vilib>:"Stop.vi"("Plan Enqueuer"=w456) -> ("error out"=w455:errorcluster)  [unwired: 10 in]
            n224 = local read "P0"() -> (w453:dbl)
            n225 = local read "Stab_Time"() -> (w451:dbl)
            n226 = local read "dP"() -> (w452:dbl)
            n227 = local read "N"() -> (w450:u32)
            n228 = local read "Stab_dP"() -> (w449:dbl)
            n229 = local read "Mix_RPM"() -> (w448:dbl)
            n230 = local read "Time"() -> (w447:dbl)
            n231 = call <vilib>:"Application Directory.vi"() -> ("Application Directory"=w446:path)
            n232 = Build Path(base path=w446, name or relative path="data\\pvt.cfg" ("string")) -> (appended path=w444:path)
            n233 = Bundle By Name(cluster=T18 {"P0"=1.0, "dP"=0.1, "Stab_Time"=0.0, "N"=1, "Stab_dP"=0.1, "Mix_RPM"=0.1, "Time"=0.0, "Item Names"=[]} ("Cluster"), "P0"=w453, "dP"=w452, "Stab_Time"=w451, "N"=w450, "Stab_dP"=w449, "Mix_RPM"=w448, "Time"=w447, "Item Names"=w437) -> (w442:T18)
            n234 = call <vilib>:"Open Config Data.vi"("configuration file path"=w444) -> ("refnum"=w443:T20)  [unwired: 8 in, 2 out]
            n235 = disable-structure shown="Enabled" {
              disable-tunnel: w443 -> [w475 _]
              disable-tunnel: w442 -> [w474 _]
              disable-tunnel: [w473 _] -> w441
              disable-tunnel: [w472 _] -> w440
              frame Disabled {
                n236 = call <userlib>:"Write INI Cluster__ogtk.vi"("INI Fomatted Cluster"=w474, "refnum"=w475) -> ("error out"=w473:errorcluster, "dup refnum"=w472:T20)  [unwired: 8 in]
              }
              frame Enabled {
              }
            }
            n237 = call <vilib>:"Close Config Data.vi"("error in (no error)"=w441, "refnum"=w440) -> ("error out"=w439:errorcluster)  [unwired: 8 in, 1 out]
            n238 = Merge Errors(w436, w439, w455, w469, w466) -> (w468:errorcluster)
          }
          frame Default {
            # "'Default' case only runs if there is a message that isn't defined in any of the other cases.  Output a programming error."
            n239 = call "Module Name--constant.vi"() -> ("Module Name"=w476:string)  [unwired: 11 in]
            n240 = xnode "Error Ring"("parameter 0"=w477, "parameter 1"=w476) -> ("error out"=w481:errorcluster)
            n241 = Merge Errors(w479, w481) -> (w480:errorcluster)
          }
        }
        n242 = call-dynamic "Delacor_lib_QMH_Error Handler - Message Handling Loop.vi"("error in"=w152, "Message Queue in"=w142) -> ("dup error in"=w149:errorcluster)  [unwired: 8 in, 1 out]
      }
    }
    frame Error {
      # "Synchronize Caller Events.vi will inform Start Module.vi that the module has launched and will let the code calling Start Module.vi register for broadcasts and would permit the caller receive the broadcast that an error occurred at launch time."
      n243 = call-dynamic "Delacor_lib_QMH_Release Message Queue.vi"("error in"=w492, "Message Queue"=w490) -> ("error out"=w491:errorcluster)  [unwired: 9 in]
      n244 = call "Synchronize Caller Events.vi"("Singleton Module Admin in"=w493) -> ("error out"=w498:errorcluster)  [unwired: 9 in, 1 out]
      n245 = call "Module Name--constant.vi"() -> ("Module Name"=w496:string)  [unwired: 11 in]
      n246 = Format Into String(format string="An error occurred during initialization. %s is no longer running.", w496) -> (resulting string=w494:string)  [unwired: 2 in, 1 out]
      n247 = Merge Errors(w491, w498) -> (w499:errorcluster)
      n248 = call "Error Reported.vi"("Additional Information"=w494, "Error"=w499) -> ()  [unwired: 9 in, 1 out]
    }
  }
  n249 = while {
    tunnel: w16 -> [w505]
    tunnel: w15 -> [w504]
    tunnel: [w503] -> w14
    tunnel: w3 -> [w500]
    stop <- w501 stop-if-true
    n250 = event shown="[0] Timeout" {
      selector: w505 -> [_ _ _]
      dyn-events: _ -> [_ _ _]
      timeout: 100 -> [_ _ _]
      tunnel: w504 -> [w510 w654 w658]
      tunnel: [w511 w653 w658] -> w503
      tunnel: [_ _ TRUE] -> w501
      tunnel: w500 -> [w506 _ _]
      event Timeout {
        # "Working Zone"
        n251 = event-data() -> ()  [unwired: 1 in, 1 out]
        n252 = local read "N 2"() -> (w507:u32)
        n253 = call "Get_Order.vi"("Control in"=w510) -> ("timed out?"=w508:bool, "Control out"=w509:T7)  [unwired: 17 in]
        n254 = case shown="False" w508 {
          tunnel: w509 -> [w517 w651]
          tunnel: [w518 w651] -> w511
          tunnel: w507 -> [w513 _]
          tunnel: w506 -> [w512 _]
          frame False {
            # "Timeout Queue"
            n255 = call "Step.vi"("Control in"=w517) -> ("Init?"=w514:bool, "Name"=w515:string, "Control out"=w516:T7)  [unwired: 16 in]
            n256 = case shown="\"Wait_Time\"" w515 {
              tunnel: w516 -> [w525 w546 w578 w607 w639 w650]
              tunnel: w514 -> [w526 w547 w579 w608 w640 _]
              tunnel: [w524 w545 w577 w606 w638 w650] -> w518
              tunnel: w513 -> [_ w541 _ w597 w632 _]
              tunnel: w512 -> [_ w538 _ w593 _ _]
              frame "Start" {
                # "Step"
                n257 = case shown="True" w526 {
                  selector: w526 -> [w531 w536]
                  tunnel: [w532 w537] -> w521
                  tunnel: w525 -> [w532 w537]
                  tunnel: [w531 w536] -> w519
                  frame False {
                  }
                  frame True {
                    # "Input Move"
                    n258 = call "Update List UI.vi"() -> ()  [unwired: 11 in, 1 out]
                    n259 = local write "N 2"(u32 1 ("N 2")) -> ()
                    n260 = call "Write_Dot.vi"("Finish?"=FALSE, "Clean?"=TRUE) -> ()  [unwired: 9 in, 1 out]
                  }
                }
                n261 = call "Timer.vi"("Control in"=w521) -> ("Timeout"=w520:dbl, "Control out"=w522:T7)  [unwired: 17 in]
                n262 = call "Timeout.vi"("Timeout"=w520, "RST"=w519) -> ("Done"=w523:bool)  [unwired: 16 in, 1 out]
                n263 = case shown="True" w523 {
                  tunnel: [w527 w529] -> w524
                  tunnel: w522 -> [w527 w530]
                  frame False {
                  }
                  frame True {
                    # "Exit Move"
                    n264 = call "BackTo.vi"("Control in"=w530, "Back Step?"="" ("Step")) -> ("Control out"=w529:T7)  [unwired: 17 in]
                  }
                }
              }
              frame "Set_P0" {
                # "Step"
                n265 = case shown="True" w547 {
                  selector: w547 -> [w552 w563]
                  tunnel: [w553 w564] -> w543
                  tunnel: w546 -> [w553 w564]
                  tunnel: [w552 w563] -> w542
                  tunnel: w541 -> [_ w562]
                  tunnel: w538 -> [_ w558]
                  frame False {
                  }
                  frame True {
                    # "Input Move"
                    n266 = property class="LstBox (strict)"(reference=w558) -> ("Item Names"=w557:string[])  [unwired: 1 in, 2 out]
                    n267 = Decrement(x=w562) -> (x-1=w556:u32)
                    n268 = Index Array(array=w557, index=w556) -> (element=w555:string)
                    n269 = Fract/Exp String To Number(string=w555) -> (number=w554:dbl)  [unwired: 3 in, 1 out]
                    "dP 2" <- w554
                    n270 = call "Update List UI.vi"() -> ()  [unwired: 11 in, 1 out]
                    n271 = call "Start_Mix.vi"("Start"=TRUE, "RPM"="Mix_RPM") -> ()  [unwired: 9 in, 1 out]
                    n272 = call "Start_Pressure.vi"("Start"=TRUE, "Pressure"=w554) -> ()  [unwired: 9 in, 1 out]
                    "Mix_RPM 2" <- "Mix_RPM"
                  }
                }
                n273 = call "Timer.vi"("Control in"=w543) -> ("Timeout"=w540:dbl, "Control out"=w544:T7)  [unwired: 17 in]
                n274 = call "Timeout.vi"("Timeout"=w540, "RST"=w542) -> ("Done"=w539:bool)  [unwired: 16 in, 1 out]
                n275 = case shown="True" w539 {
                  tunnel: [w548 w550] -> w545
                  tunnel: w544 -> [w548 w551]
                  frame False {
                  }
                  frame True {
                    # "Exit Move"
                    n276 = call "BackTo.vi"("Control in"=w551, "Back Step?"="" ("Step")) -> ("Control out"=w550:T7)  [unwired: 17 in]
                  }
                }
              }
              frame "Wait_Stab" {
                # "Step"
                n277 = case shown="True" w579 {
                  selector: w579 -> [w587 w590]
                  tunnel: [w588 w591] -> w575
                  tunnel: w578 -> [w588 w591]
                  tunnel: [w587 w590] -> w574
                  tunnel: [w586 w589] -> w568
                  frame False {
                    n278 = local read "relative seconds"() -> (w586:dbl)
                  }
                  frame True {
                    # "Input Move"
                    n279 = call <vilib>:"High Resolution Relative Seconds.vi"() -> ("relative seconds"=w589:dbl)
                    "relative seconds" <- w589
                  }
                }
                n280 = call <vilib>:"High Resolution Relative Seconds.vi"() -> ("relative seconds"=w569:dbl)
                n281 = local read "Stab_dP 2"() -> (w573:dbl)
                n282 = Subtract(x=w569, y=w568) -> (x-y=w565:dbl)
                "Stab_Time 2" <- w565
                n283 = Less?(x=w573, y="Stab_dP") -> (x < y?=w571:bool)
                n284 = Less Or Equal?(x="Stab_Time", y=w565) -> (x <= y?=w566:bool)
                n285 = call "Timer.vi"("Control in"=w575) -> ("Control out"=w576:T7)  [unwired: 17 in, 1 out]
                n286 = call "Timeout.vi"("Timeout"="Stab_Time", "RST"=w574) -> ()  [unwired: 16 in, 2 out]
                n287 = And(x=w566, y=w571) -> (x .and. y?=w570:bool)
                n288 = case shown="True" w570 {
                  tunnel: [w580 w584] -> w577
                  tunnel: w576 -> [w580 w585]
                  frame False {
                  }
                  frame True {
                    w581 = 0.0 ("RPM")
                    # "Мешалка выкл"
                    # "Exit Move"
                    n289 = local write "Mix_RPM 2"(w581) -> ()
                    n290 = call "Start_Mix.vi"("Start"=FALSE, "RPM"=w581) -> ()  [unwired: 9 in, 1 out]
                    n291 = call "BackTo.vi"("Control in"=w585, "Back Step?"="" ("Step")) -> ("Control out"=w584:T7)  [unwired: 17 in]
                  }
                }
              }
              frame "Wait_Time" {
                # "Step"
                n292 = case shown="True" w608 {
                  selector: w608 -> [w628 w630]
                  tunnel: [w629 w631] -> w603
                  tunnel: w607 -> [w629 w631]
                  tunnel: [w628 w630] -> w602
                  frame False {
                  }
                  frame True {
                    # "Input Move"
                  }
                }
                n293 = property class="LstBox (strict)"(reference=w593) -> ("Item Names"=w596:string[])  [unwired: 1 in, 2 out]
                n294 = Index Array(array=w596, index=0) -> (element=w595:string)
                n295 = Fract/Exp String To Number(string=w595) -> (number=w592:dbl)  [unwired: 3 in, 1 out]
                n296 = call "Timer.vi"("Control in"=w603) -> ("Control out"=w604:T7)  [unwired: 17 in, 1 out]
                n297 = Greater?(x="N", y=w597) -> (0:w598:bool)
                n298 = call "Timeout.vi"("Timeout"="Time", "RST"=w602) -> ("dT"=→"Time 2":dbl, "Done"=w605:bool)  [unwired: 16 in]
                n299 = case shown="True" w605 {
                  tunnel: [w609 w619] -> w606
                  tunnel: w604 -> [w609 w620]
                  tunnel: w598 -> [_ w617]
                  tunnel: w598 -> [_ w612]
                  tunnel: w597 -> [_ w614]
                  tunnel: w592 -> [_ w610]
                  frame False {
                  }
                  frame True {
                    # "Exit Move"
                    n300 = case shown="False" w612 {
                      tunnel: w614 -> [_ w626]
                      tunnel: w610 -> [w623 _]
                      frame False {
                        # "Мешалка выкл"
                        n301 = local read "Mix_RPM"() -> (w621:dbl)
                        n302 = local write "Mix_RPM 2"(w621) -> ()
                        n303 = local write "dP 2"(w623) -> ()
                        n304 = call "Start_Mix.vi"("Start"=TRUE, "RPM"=w621) -> ()  [unwired: 9 in, 1 out]
                        n305 = local write "N 2"(u32 1 ("N 2")) -> ()
                        n306 = call "Update List UI.vi"() -> ()  [unwired: 11 in, 1 out]
                        n307 = call "Start_Pressure.vi"("Start"=TRUE, "Pressure"=w623) -> ()  [unwired: 9 in, 1 out]
                      }
                      frame True {
                        n308 = Increment(x=w626) -> (x+1=→"N 2":u32)
                      }
                    }
                    n309 = Not(x=w612) -> (.not. x?=w611:bool)
                    n310 = Select(t="Set_P0", s=w617, f="" ("Step")) -> (s? t:f=w618:string)
                    n311 = call "BackTo.vi"("Control in"=w620, "Back Step?"=w618) -> ("Control out"=w619:T7)  [unwired: 17 in]
                    n312 = call "Write_Dot.vi"("Finish?"=w611, "Clean?"=FALSE) -> ()  [unwired: 9 in, 1 out]
                  }
                }
              }
              frame "Inc" {
                # "Step"
                n313 = case shown="True" w640 {
                  selector: w640 -> [w645 w647]
                  tunnel: [w646 w648] -> w635
                  tunnel: w639 -> [w646 w648]
                  tunnel: [w645 w647] -> w633
                  tunnel: w632 -> [_ _]
                  frame False {
                  }
                  frame True {
                    # "Input Move"
                  }
                }
                n314 = call "Timer.vi"("Control in"=w635) -> ("Timeout"=w634:dbl, "Control out"=w636:T7)  [unwired: 17 in]
                n315 = call "Timeout.vi"("Timeout"=w634, "RST"=w633) -> ("Done"=w637:bool)  [unwired: 16 in, 1 out]
                n316 = case shown="True" w637 {
                  tunnel: [w641 w643] -> w638
                  tunnel: w636 -> [w641 w644]
                  frame False {
                  }
                  frame True {
                    # "Exit Move"
                    n317 = call "BackTo.vi"("Control in"=w644, "Back Step?"="" ("Step")) -> ("Control out"=w643:T7)  [unwired: 17 in]
                  }
                }
              }
              frame "Stop", Default {
                n318 = local write "Start"(FALSE ("Start")) -> ()
              }
            }
          }
          frame True {
          }
        }
      }
      event "Start": Value Change {
        # "Event Start-Stop Cycle"
        n319 = event-data() -> ("NewVal"=w652:bool)  [unwired: 1 in]
        n320 = case shown="False" w652 {
          frame False {
            n321 = call "Write_Dot.vi"("Finish?"=TRUE, "Clean?"=FALSE) -> ()  [unwired: 9 in, 1 out]
          }
          frame True {
          }
        }
        n322 = call <vilib>:"Start.vi"("On/Off"=w652, "Control in"=w654) -> ("Control out"=w653:T7)  [unwired: 17 in]
      }
      event User Event {
        # "Exit event"
        n323 = event-data() -> ()  [unwired: 1 in, 1 out]
      }
    }
  }
  n324 = Merge Errors(w29, w32) -> (w28:errorcluster)
  n325 = call "Close Module.vi"("error in (no error)"=w28, "Module Admin in"=w23) -> ("error out"=w30:errorcluster, "External Launch"=w17:bool, "Module Admin out"=w18:refnum<class "Delacor_lib_QMH_Module Admin.lvclass">)  [unwired: 7 in]
  n326 = Unregister For Events(event registration refnum=w22, error in=w30) -> (error out=w27:errorcluster)
  "error out" <- w27
  n327 = call "Destroy.vi"("Control"=w14) -> ()  [unwired: 19 in]
  n328 = case "External Launch?" shown="True" w17 {
    tunnel: w27 -> [_ w659]
    frame False {
    }
    frame True {
      n329 = case shown="Error" w659 {
        frame No Error {
          n330 = invoke class="VI" method="FP.Close"() -> ()  [unwired: 3 in, 3 out]
        }
        frame Error {
          n331 = disable-structure shown="Disabled" {
            frame Disabled {
              n332 = invoke class="VI" method="FP.Open"("Activate"=TRUE ("Activate?")) -> ()  [unwired: 4 in, 5 out]
            }
            frame Enabled {
            }
          }
        }
      }
    }
  }
  n333 = local write "Module Admin"(w18) -> ()
  n334 = disable-structure shown="Disabled" {
    frame Disabled {
      n335 = event "DQMH_EVENT_MAIN" shown="[6] <Drive Broadcast Events.Pump_Data>: User Event" {
        selector: _ -> [_ _ _ _ _ _ _ _ _ _ _ _ _ _ _ _ _ _ _ _ _]
        dyn-events: _ -> [_ _ _ _ _ _ _ _ _ _ _ _ _ _ _ _ _ _ _ _ _]
        timeout: _ -> [_ _ _ _ _ _ _ _ _ _ _ _ _ _ _ _ _ _ _ _ _]
        tunnel: [_ _ _ _ TRUE ("Discard?") _ _ _ _ _ _ _ _ _ _ _ _ _ _ _ _] -> _
        tunnel: _ -> [_ _ _ _ w682 w689 w700 w708 _ w725 w729 w731 w734 w737 w740 w744 w748 w754 _ w762 w763]
        tunnel: [_ _ w666 _ w685 w691 w701 w703 w709 w722 w726 w732 w735 w738 w741 w745 _ w749 w756 w757 w764] -> _
        tunnel: _ -> [_ _ _ _ _ w688 _ _ _ _ _ _ _ _ _ _ _ _ _ _ _]
        event User Event {
          # "Show the panel of this VI, and send a status updated message to let listeners know."
          # "Another Module called the \"Show Panel\" API Method."
          n336 = event-data() -> ()  [unwired: 1 in, 1 out]
          n337 = control-ref of="This VI"() -> (w662:refnum<vi>)
          n338 = call "Open VI Panel.vi"("VI"=w662) -> ()  [unwired: 10 in, 1 out]
          n339 = call "Status Updated.vi"("Status"="Panel shown." ("format string")) -> ()  [unwired: 10 in, 1 out]
        }
        event User Event {
          # "Hide the panel of this VI, and send a status updated message to let listeners know."
          # "Another Module called the \"Hide Panel\" API Method."
          n340 = event-data() -> ()  [unwired: 1 in, 1 out]
          n341 = control-ref of="This VI"() -> (w664:refnum<vi>)
          n342 = call "Hide VI Panel.vi"("VI"=w664) -> ()  [unwired: 10 in, 1 out]
          n343 = call "Status Updated.vi"("Status"="Panel hidden." ("format string")) -> ()  [unwired: 10 in, 1 out]
        }
        event User Event {
          # "Another Module called the \"Get Module Execution Status\" API Method."
          n344 = event-data() -> ()  [unwired: 1 in, 1 out]
          n345 = call "Update Module Execution Status.vi"("Running?"=TRUE) -> ("error out"=w666:errorcluster)  [unwired: 10 in]
        }
        event User Event {
          # "Another Module called the \"Show Diagram\" API Method. This event is used for debugging."
          n346 = event-data() -> ()  [unwired: 1 in, 1 out]
          n347 = disable-structure shown="RUN_TIME_ENGINE==False" {
            frame condition #0 (active) {
              # "functionality not available in exe"
              n348 = invoke class="VI" method="Lock State.Get"() -> (error out=w672:errorcluster, "Get Lock State"=w671:T13, "pwd in cache"=w668:bool)  [unwired: 4 in, 1 out]
              n349 = Equal?(x=T13."Password-protected", y=w671) -> (x = y?=w669:bool)
              n350 = Compound Arithmetic op=AND(w669, invert w668) -> (w667:bool)
              n351 = case shown="False" w667 {
                tunnel: w672 -> [w675 _]
                frame False {
                  n352 = property class="VI"(error in=w675, "BDWin.Open"=TRUE ("Block Diagram Window:Open")) -> ()  [unwired: 1 in, 2 out]
                  n353 = call "Status Updated.vi"("Status"="Block Diagram shown." ("format string")) -> ()  [unwired: 10 in, 1 out]
                }
                frame True {
                  # "Password-protected VI, and the password is not in the cache. Do not show the diagram."
                }
              }
            }
            frame condition #1 {
            }
          }
        }
        event User Event {
          # "The Stop Module Event can get fired from the Exit message in the MHL. The queue gets destroyed in that case. If the queue no longer exists, the Enqueue Exit as a priority message will return error 1. It is safe to ignore, because the module is already exiting."
          # "Another Module called the \"Stop Module\" API Method  or the Message Handling Loop below."
          n354 = event-data() -> ("Exit via Stop Module Req?"=w678:bool, "Wait for Module to stop?"=w677:bool)  [unwired: 1 in, 1 out]
          n355 = Bundle By Name(cluster=T14 {"Origin"="", "Exit via Stop Module Req?"=FALSE, "Wait for Module to stop?"=FALSE} ("Stop Argument"), "Exit via Stop Module Req?"=w678, "Wait for Module to stop?"=w677) -> (w676:T14)
          n356 = call-poly <vilib>:"Delacor_lib_QMH_Enqueue Message (poly).vi"("Priority Message? (F)"=TRUE, "Message Data"=w676, "Message"="Exit", "Message Queue in"=w682) -> ("error out"=w686:errorcluster)  [unwired: 6 in, 1 out]
          n357 = call <vilib>:"Clear Errors.vi"("error in (no error)"=w686, "specific error code to clear (0: all)"=1) -> ("error out"=w685:errorcluster)  [unwired: 4 in, 1 out]
        }
        event Panel Close? {
          w690 = TRUE  # Discard the event, the MHL is responsible for closing and stopping this VI.
          # "Hide the panel or send the 'Exit' message if the user clicks the 'X' on the module main VI panel."
          n358 = event-data() -> ()  [unwired: 1 in, 1 out]
          n359 = property class="Module Admin"(reference=w688) -> ("Accessors:External Launch"=w687:bool)  [unwired: 1 in, 2 out]
          n360 = case shown="False" w687 {
            tunnel: w689 -> [_ w695]
            tunnel: [_ w696] -> w691
            frame True {
              # "If externally launched, clicking the 'X' hides the panel, but doesn't close it."
              n361 = control-ref of="This VI"() -> (w692:refnum<vi>)
              n362 = call "Hide VI Panel.vi"("VI"=w692) -> ()  [unwired: 10 in, 1 out]
            }
            frame False {
              # "If run as a stand-alone VI, clicking the panel 'X' stops the VI."
              n363 = call-poly <vilib>:"Delacor_lib_QMH_Enqueue Message (poly).vi"("Priority Message? (F)"=TRUE, "Message"="Exit", "Message Queue in"=w695) -> ("error out"=w696:errorcluster)  [unwired: 7 in, 1 out]
            }
          }
          n364 = event-data("Discard?"=w690) -> ()  [unwired: 1 in, 1 out]
        }
        event User Event {
          n365 = event-data() -> ("Pump_data"=w699:T10)  [unwired: 1 in]
          n366 = To Variant(anything=w699) -> (Variant=w697:variant)
          n367 = call-poly <vilib>:"Delacor_lib_QMH_Enqueue Message (poly).vi"("Message Data"=w697, "Message"="Drive_Data", "Message Queue in"=w700) -> ("error out"=w701:errorcluster)  [unwired: 7 in, 1 out]
        }
        event User Event {
          # "Another Module called the \"Write_Dot\" API Method."
          n368 = event-data() -> ("Clean?"=w704:bool, "Finish?"=w702:bool)  [unwired: 1 in]
          n369 = Bundle(cluster=T15 {"Clean?"=FALSE, "Finish?"=FALSE} ("Write_Dot Argument"), "Clean?"=w704, "Finish?"=w702) -> (w705:T15)
          n370 = call-poly <vilib>:"Delacor_lib_QMH_Enqueue Message (poly).vi"("Message Data"=w705, "Message"="Write_Dot", "Message Queue in"=w708) -> ("error out"=w703:errorcluster)  [unwired: 7 in, 1 out]
        }
        event #8 (no event record) {
          w713 = "\""
          w721 = T21 2 items=["User Home"=0, "User Desktop"=1, "User Documents"=2, "User Application Data"=3, "User Preferences"=4, "User Temporary"=5, "Public Documents"=6, "Public Application Data"=7, "Public Preferences"=8, "Public Cache"=13, "System Core Libraries"=9, "System Installed Libraries"=10, "Application Files"=11, "Boot Volume Root"=12] ("system directory type")
          n371 = event-data() -> ()  [unwired: 1 in, 6 out]
          n372 = call <vilib>:"Get System Directory.vi"("system directory type"=w721) -> ("system directory"=w720:path)  [unwired: 10 in]
          n373 = Build Path(base path=w720, name or relative path="PVT") -> (appended path=w717:path)
          n374 = Create Folder(path (use dialog)=w717) -> (created path=w711:path, error out=w718:errorcluster)  [unwired: 2 in, 1 out]
          n375 = call <vilib>:"Clear Errors.vi"("error in (no error)"=w718) -> ("error out"=w710:errorcluster)  [unwired: 5 in, 1 out]
          n376 = Path To String(path=w711) -> (string=w714:string)
          n377 = Concatenate Strings(w713, w714, w713) -> (w712:string)
          n378 = Concatenate Strings("explorer.exe " ("command line"), w712) -> (w715:string)
          n379 = call <vilib>:"System Exec.vi"("error in (no error)"=w710, "command line"=w715) -> ("error out"=w709:errorcluster)  [unwired: 6 in, 3 out]
        }
        event User Event {
          n380 = event-data() -> ("Исходные данные"=w724:T11)  [unwired: 1 in]
          n381 = call-poly <vilib>:"Delacor_lib_QMH_Enqueue Message (poly).vi"("Message Data"=w724, "Message"="Initial Data", "Message Queue in"=w725) -> ("error out"=w722:errorcluster)  [unwired: 7 in, 1 out]
        }
        event User Event {
          n382 = event-data() -> ("Temp array"=w728:dbl[])  [unwired: 1 in]
          n383 = call-poly <vilib>:"Delacor_lib_QMH_Enqueue Message (poly).vi"("Message Data"=w728, "Message"="Temp Data", "Message Queue in"=w729) -> ("error out"=w726:errorcluster)  [unwired: 7 in, 1 out]
        }
        event "Load": Value Change {
          n384 = event-data() -> ()  [unwired: 1 in, 1 out]
          n385 = call-poly <vilib>:"Delacor_lib_QMH_Enqueue Message (poly).vi"("Message"="Load List", "Message Queue in"=w731) -> ("error out"=w732:errorcluster)  [unwired: 8 in, 1 out]
        }
        event "Save": Value Change {
          n386 = event-data() -> ()  [unwired: 1 in, 1 out]
          n387 = call-poly <vilib>:"Delacor_lib_QMH_Enqueue Message (poly).vi"("Message"="Save List", "Message Queue in"=w734) -> ("error out"=w735:errorcluster)  [unwired: 8 in, 1 out]
        }
        event "Delete": Value Change {
          n388 = event-data() -> ()  [unwired: 1 in, 1 out]
          n389 = call-poly <vilib>:"Delacor_lib_QMH_Enqueue Message (poly).vi"("Message"="Delete Row", "Message Queue in"=w737) -> ("error out"=w738:errorcluster)  [unwired: 8 in, 1 out]
        }
        event "Add": Value Change {
          n390 = event-data() -> ()  [unwired: 1 in, 1 out]
          n391 = call-poly <vilib>:"Delacor_lib_QMH_Enqueue Message (poly).vi"("Message"="Add Row", "Message Queue in"=w740) -> ("error out"=w741:errorcluster)  [unwired: 8 in, 1 out]
        }
        event "Pressure_List": Value Change {
          n392 = event-data() -> ("NewVal"=w743:i32)  [unwired: 1 in]
          n393 = call-poly <vilib>:"Delacor_lib_QMH_Enqueue Message (poly).vi"("Message Data"=w743, "Message"="Select Row", "Message Queue in"=w744) -> ("error out"=w745:errorcluster)  [unwired: 7 in, 1 out]
        }
        event "Pressure_edit": Value Change {
          n394 = event-data() -> ("NewVal"=w747:dbl)  [unwired: 1 in]
          n395 = call-poly <vilib>:"Delacor_lib_QMH_Enqueue Message (poly).vi"("Message Data"=w747, "Message"="Value change", "Message Queue in"=w748) -> ()  [unwired: 7 in, 2 out]
        }
        event User Event {
          # "Another Module called the \"Update List UI\" API Method."
          n396 = event-data() -> ("Boolean"=w750:bool)  [unwired: 1 in]
          n397 = Bundle(cluster=T16 {"Boolean"=FALSE} ("Update List UI Argument"), "Boolean"=w750) -> (w751:T16)
          n398 = call-poly <vilib>:"Delacor_lib_QMH_Enqueue Message (poly).vi"("Message Data"=w751, "Message"="Update List UI", "Message Queue in"=w754) -> ("error out"=w749:errorcluster)  [unwired: 7 in, 1 out]
        }
        event User Event {
          n399 = event-data() -> ()  [unwired: 1 in, 5 out]
          n400 = property on="Start" class="Bool (strict)"("Val(Sgnl)"=FALSE ("Value (Signaling)")) -> (error out=w756:errorcluster)  [unwired: 2 in, 1 out]
        }
        event User Event {
          # "Another Module called the \"SubPanel\" API Method."
          n401 = event-data() -> ("Sub Panel"=w758:refnum<vi>)  [unwired: 1 in]
          n402 = Bundle(cluster=T17 {"Sub Panel"=refnum} ("SubPanel Argument"), "Sub Panel"=w758) -> (w759:T17)
          n403 = call-poly <vilib>:"Delacor_lib_QMH_Enqueue Message (poly).vi"("Message Data"=w759, "Message"="SubPanel", "Message Queue in"=w762) -> ("error out"=w757:errorcluster)  [unwired: 7 in, 1 out]
        }
        event "Pop-Out Tool": Value Change {
          n404 = event-data() -> ()  [unwired: 1 in, 2 out]
          n405 = call-poly <vilib>:"Delacor_lib_QMH_Enqueue Message (poly).vi"("Message"="Window", "Message Queue in"=w763) -> ("error out"=w764:errorcluster)  [unwired: 8 in, 1 out]
        }
      }
    }
    frame Enabled {
    }
  }
